vi "Reply (message).vi"(8 "error in (no error)":errorcluster, 10 "Reply":refnum<class "MSG.lvclass">, 11 "Message to Reply to":refnum<class "MSG.lvclass">) -> (0 "error out":errorcluster, 3 "Message":refnum<class "MSG.lvclass">)   [LabVIEW 2011, in "Messenging.lvlib" / "MSG.lvclass"]
uses:
  MSG.lvclass
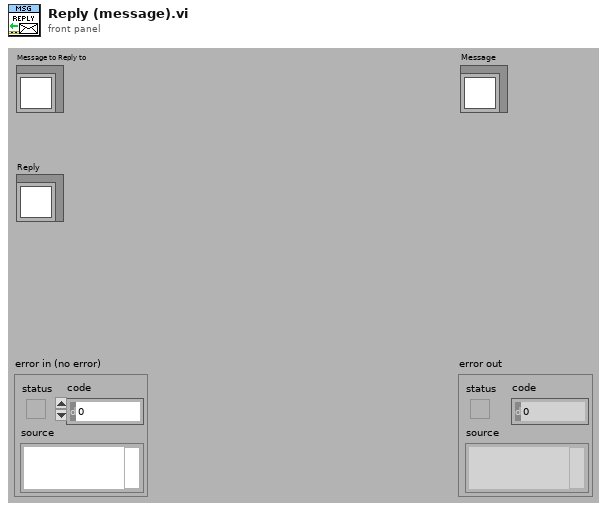
[diagram p1: front panel]
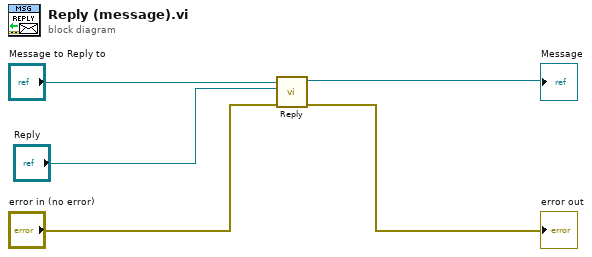
[diagram p0: block diagram]
diagram:
  n1 = call-dynamic "Reply.vi"("error in (no error)"="error in (no error)", "Reply"="Reply", "Message to Reply to"="Message to Reply to") -> ("error out"=→"error out":errorcluster, "Message"=→"Message":refnum<class "MSG.lvclass">)  [unwired: 7 out]
